vi "SmartBackground.vi"(10 "ROI":refnum<vi>, 11 "Input Graph":refnum<vi>) -> ()   [LabVIEW 2014]
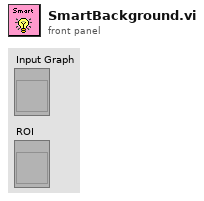
[diagram p1: front panel]
types:
  T1 = typedef "LVPointDoubleTypeDef.ctl" = cluster{"Cursor X":dbl, "Cursor Y":dbl}
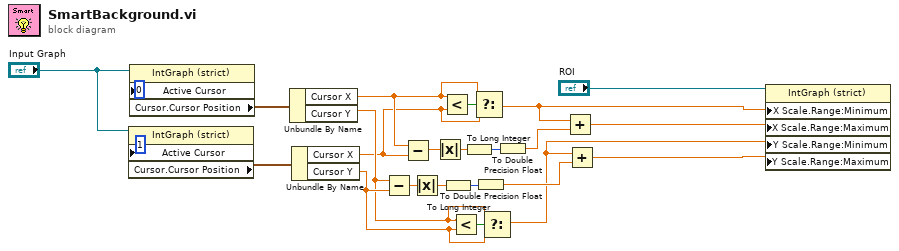
[diagram p0: block diagram]
diagram:
  n1 = property on="Property Node" class="IntGraph (strict)"(reference="Input Graph", "Active Cursor"=u32 1) -> ("Cursor.Cursor Position"=w22:T1)  [unwired: 1 in, 2 out]
  n2 = property on="Property Node" class="IntGraph (strict)"(reference="Input Graph", "Active Cursor"=u32 0) -> ("Cursor.Cursor Position"=w21:T1)  [unwired: 1 in, 2 out]
  n3 = Unbundle By Name(w21) -> ("Cursor X"=w15:dbl, "Cursor Y"=w12:dbl)
  n4 = Unbundle By Name(w22) -> ("Cursor X"=w7:dbl, "Cursor Y"=w13:dbl)
  n5 = Subtract(x=w12, y=w13) -> (x-y=w19:dbl)
  n6 = Subtract(x=w15, y=w7) -> (x-y=w20:dbl)
  n7 = Absolute Value(x=w19) -> (abs(x)=w18:dbl)
  n8 = Absolute Value(x=w20) -> (abs(x)=w17:dbl)
  n9 = Less?(x=w15, y=w7) -> (x < y?=w16:bool)
  n10 = To Long Integer(number=w18) -> (32bit integer=w9:i32)
  n11 = Less?(x=w12, y=w13) -> (x < y?=w14:bool)
  n12 = To Long Integer(number=w17) -> (32bit integer=w8:i32)
  n13 = Select(t=w15, s=w16, f=w7) -> (s? t:f=w4:dbl)
  n14 = To Double Precision Float(number=w9) -> (double precision float=w10:dbl)
  n15 = Select(t=w12, s=w14, f=w13) -> (s? t:f=w2:dbl)
  n16 = To Double Precision Float(number=w8) -> (double precision float=w11:dbl)
  n17 = Add(x=w4, y=w11) -> (x+y=w3:dbl)
  n18 = Add(x=w2, y=w10) -> (x+y=w1:dbl)
  n19 = property on="Property Node" class="IntGraph (strict)"(reference="ROI", "X Scale.Range:Minimum"=w4, "X Scale.Range:Maximum"=w3, "Y Scale.Range:Minimum"=w2, "Y Scale.Range:Maximum"=w1) -> ()  [unwired: 1 in, 2 out]
